vi "AO Post Step Type.vi"(8 "error in (no error)":errorcluster, 9 "AOWrite":T1, 10 "Socket No":u16=1, 11 "NI Analog Output in":refnum<class "NI Analog Output.lvclass">) -> (0 "error out":errorcluster, 2 "PhysicalChannel":string[](array[string]), 3 "NI Analog Output out":refnum<class "NI Analog Output.lvclass">)   [LabVIEW 2023, in "HardwareAbstractionLayer_LVOOP.lvlib" / "NI Analog Output.lvclass"]
uses:
  NI Analog Output.lvclass
  D:/eDCU LTT/VT LTT Project/Source Code/HardwareAbstractionLayer_LVOOP/Analog Output/AO/AO.lvclass
  NI Analog Output.lvclass/NI Analog Output.ctl
  Main/Class Options.ctl
  Main/Class Ref.ctl
  DMM/DMM.lvclass
  Function Generator/Function Generator.lvclass
  Oscilloscope/Oscilloscope.lvclass
  PowerSupply/PowerSupply.lvclass
  Teststand/Teststand.lvclass
  AO/AO.lvclass
  Analog Input/AI/AI.lvclass
  Database/Database.lvclass
  Digital Output/DO_class/DO.lvclass
  Digital Input/DI_class/DI.lvclass
  PWM Output/PWM Output_class/PWM Output.lvclass
  PWM Input/PWM Input_class/PWM Input.lvclass
  NI Switch/NISwitch_class/NISwitch.lvclass
  Modbus/Modbus_class/Modbus.lvclass
  CAN/CAN Lib/CAN_class/CAN.lvclass
  <resource>/objmgr/daqmx.rc
  Main/Main.lvclass
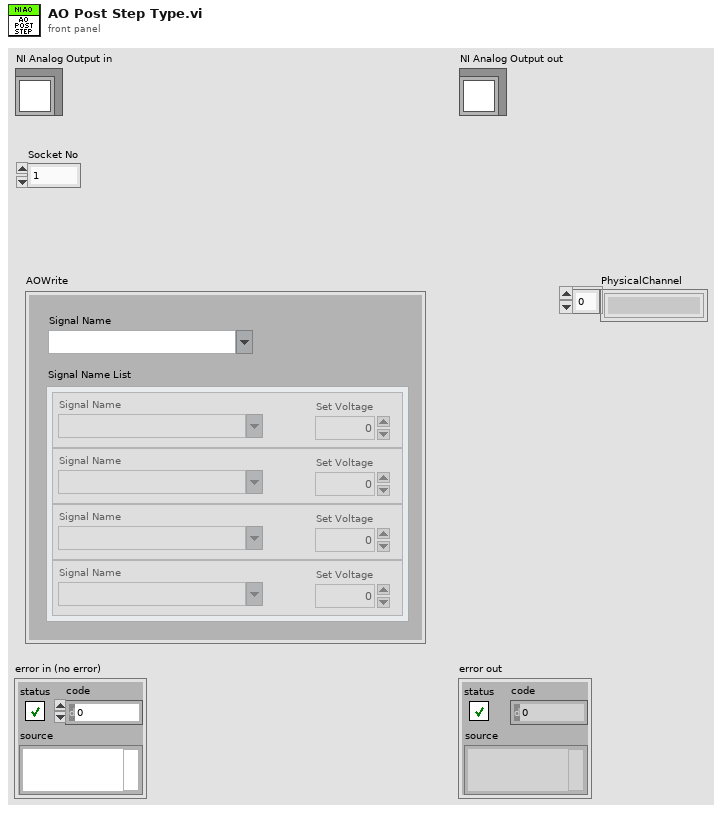
[diagram p1: front panel]
types:
  T1 = cluster{"Signal Name":string, "Signal Name List":cluster{"Signal Name":string, "Set Voltage":dbl}[]}
  T2 = typedef "HardwareAbstractionLayer_LVOOP.lvlib/Main.lvclass/Class Ref.ctl" = cluster{"DMM":refnum<class "DMM.lvclass">, "Function Generator":refnum<class "Function Generator.lvclass">, "Oscilloscope":refnum<class "Oscilloscope.lvclass">, "PowerSupply":refnum<class "PowerSupply.lvclass">, "Teststand":refnum<class "Teststand.lvclass">, "AO":refnum<class "AO.lvclass">, "AI":refnum<class "AI.lvclass">, "Database":refnum<class "Database.lvclass">, "AO Waveform Generation":refnum<class "AO.lvclass">, "DO":refnum<class "DO.lvclass">, "DI":refnum<class "DI.lvclass">, "PWM Output":refnum<class "PWM Output.lvclass">, "PWM Input":refnum<class "PWM Input.lvclass">, "RelayOutput":refnum<class "NISwitch.lvclass">, "Modbus":refnum<class "Modbus.lvclass">, "CAN":refnum<class "CAN.lvclass">}
  T3 = typedef "HardwareAbstractionLayer_LVOOP.lvlib/Main.lvclass/Class Options.ctl" = enum16{"Init All Class", "Read All Class", "Write AI Class", "Write AO Class", "Write AO Waveform Generation", "Write DI Class", "Write DO Class", "Write PWM Input Class", "Write PWM Output Class", "Exit"}
  T4 = cluster{"table":string, "condition":string, "columns":string[]}
  T5 = cluster{"Signal Name":string, "Set Voltage":dbl}[]
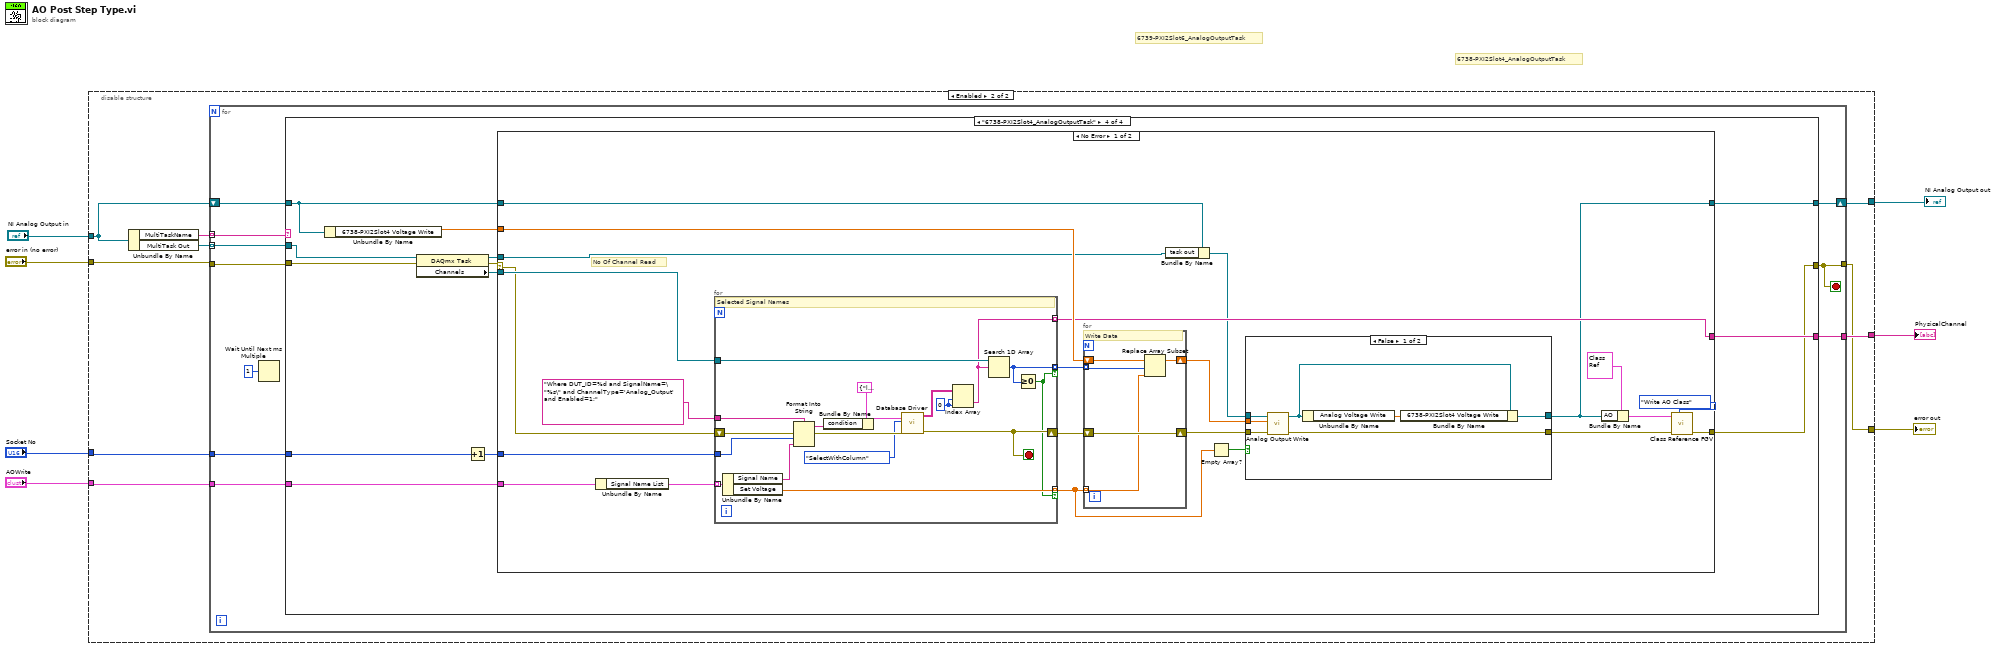
[diagram p0: block diagram]
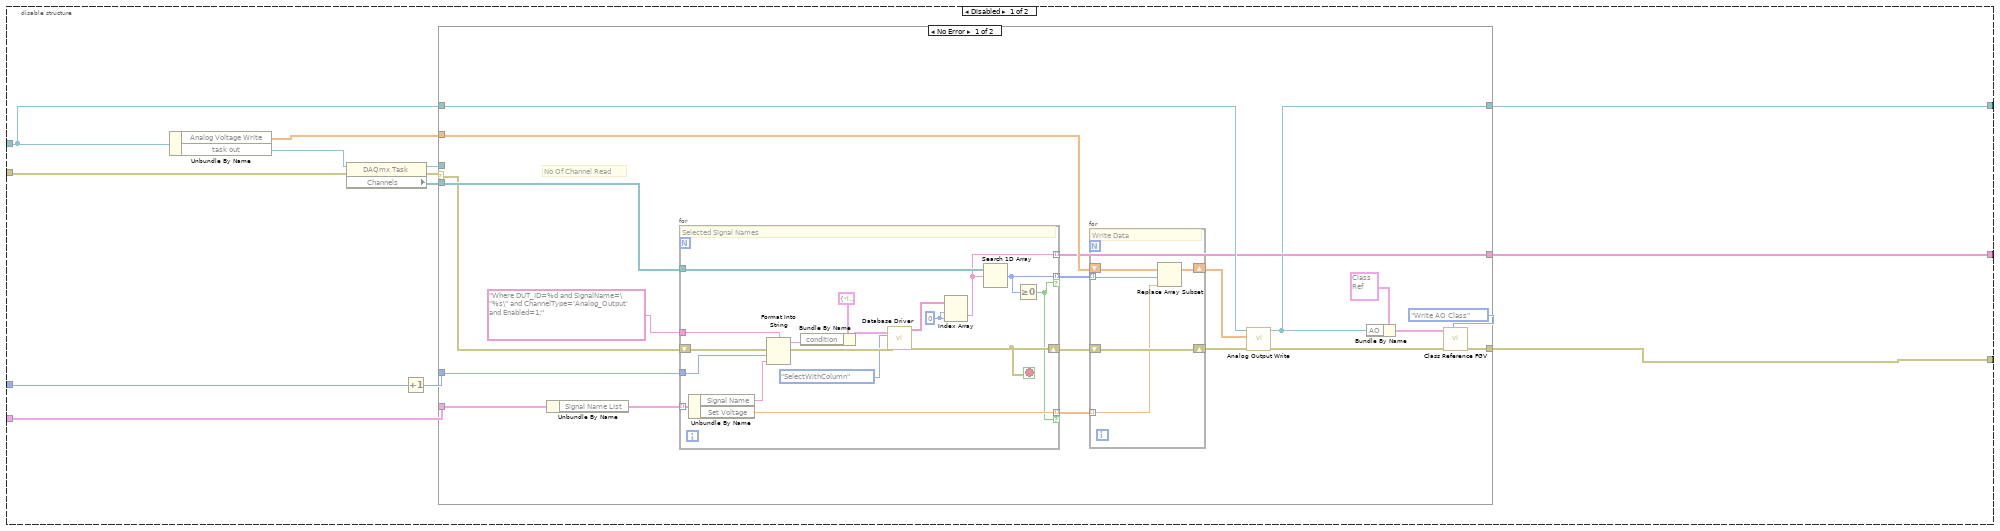
[diagram p2: hidden frame]
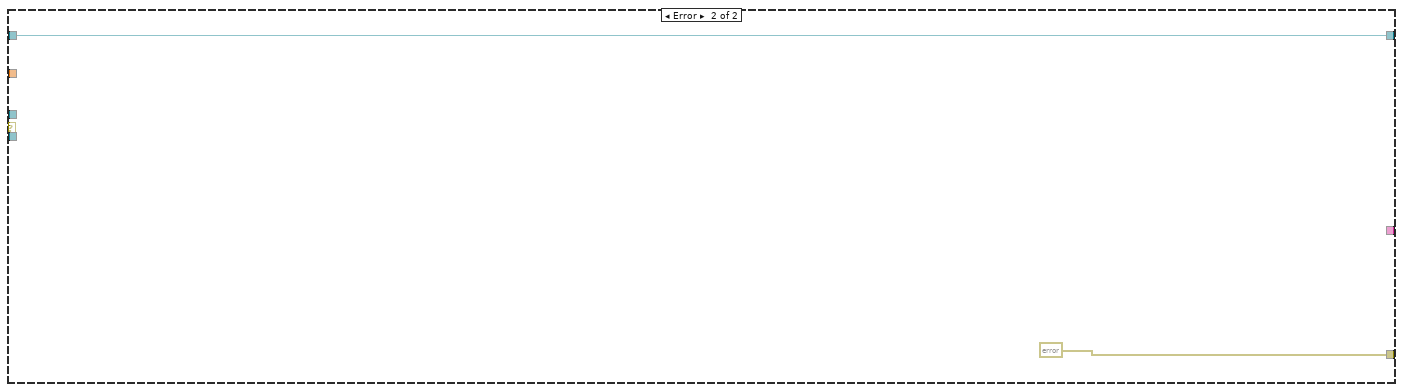
[diagram p3: hidden frame]
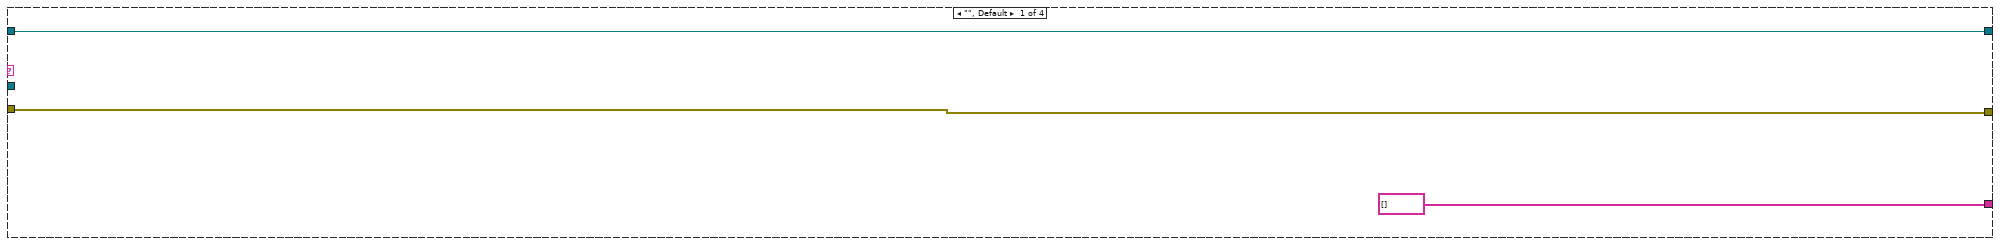
[diagram p4: hidden frame]
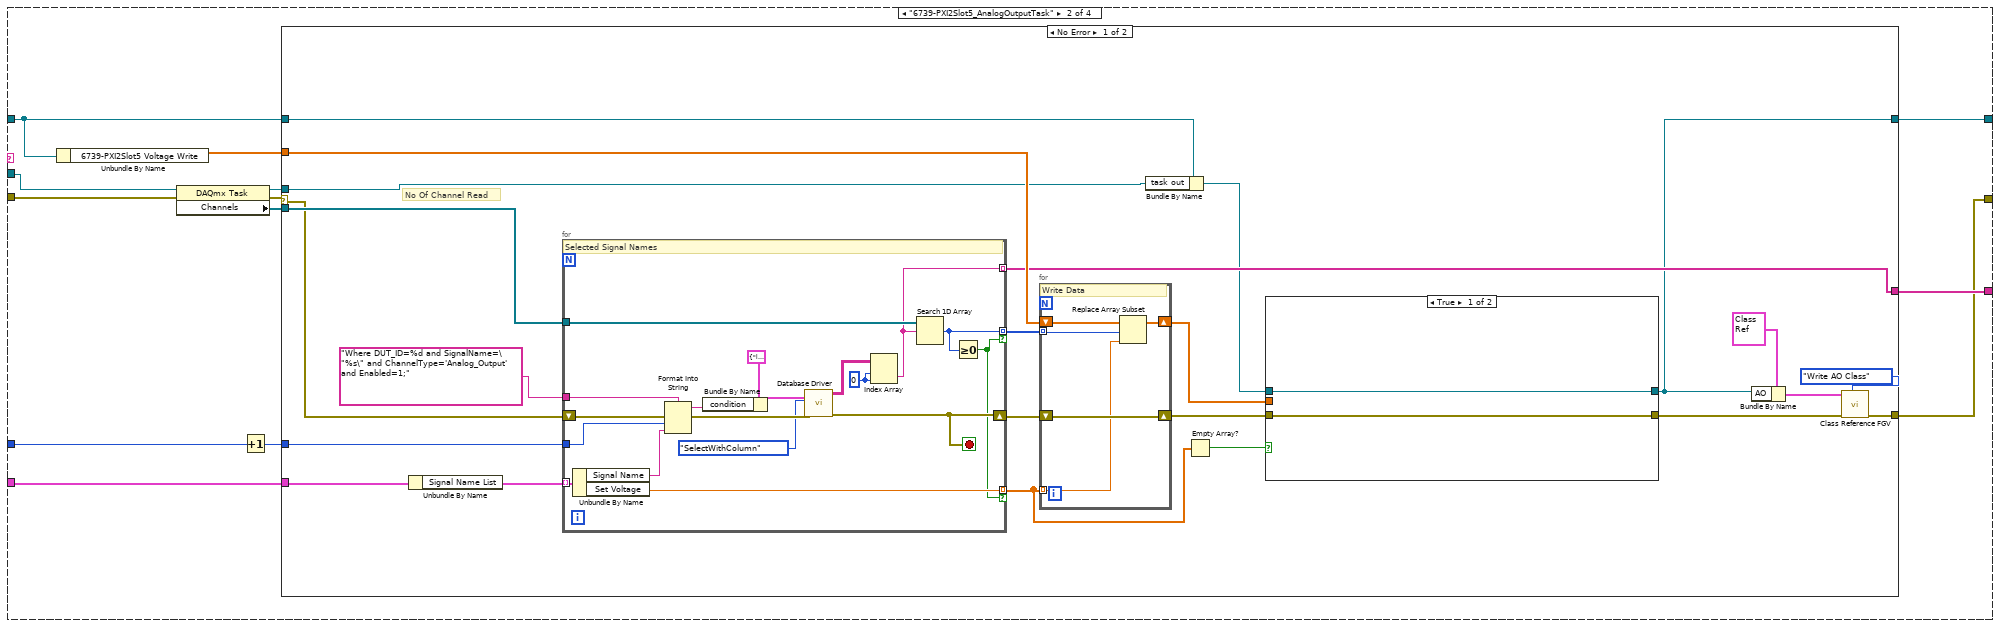
[diagram p5: hidden frame]
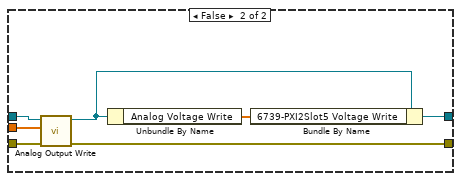
[diagram p6: hidden frame]
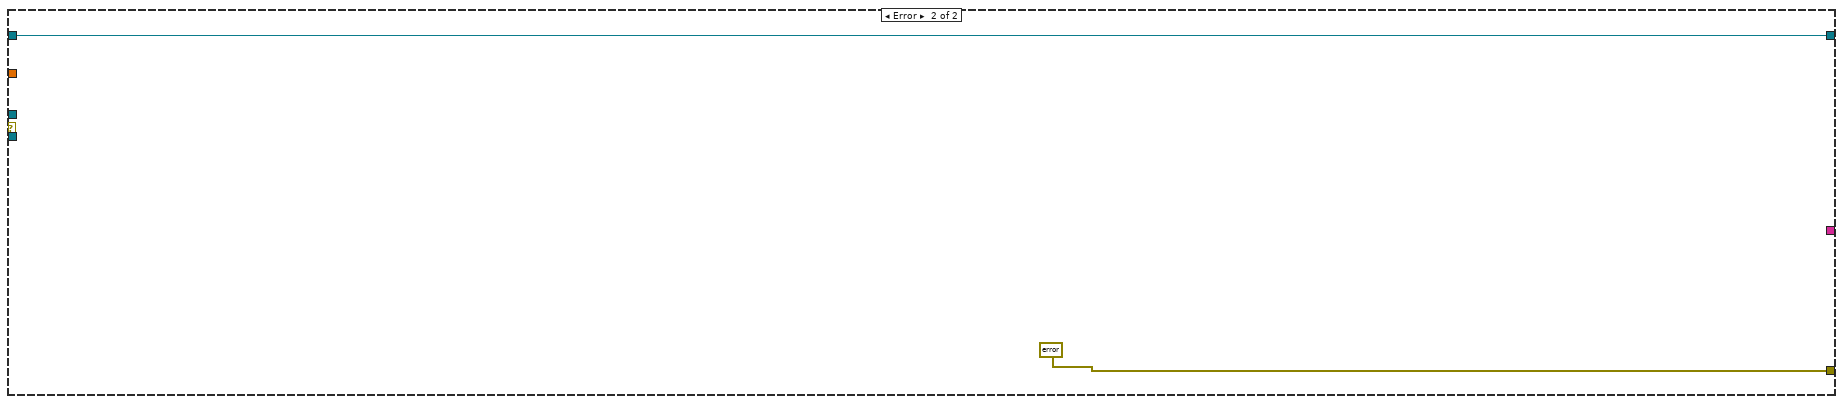
[diagram p7: hidden frame]
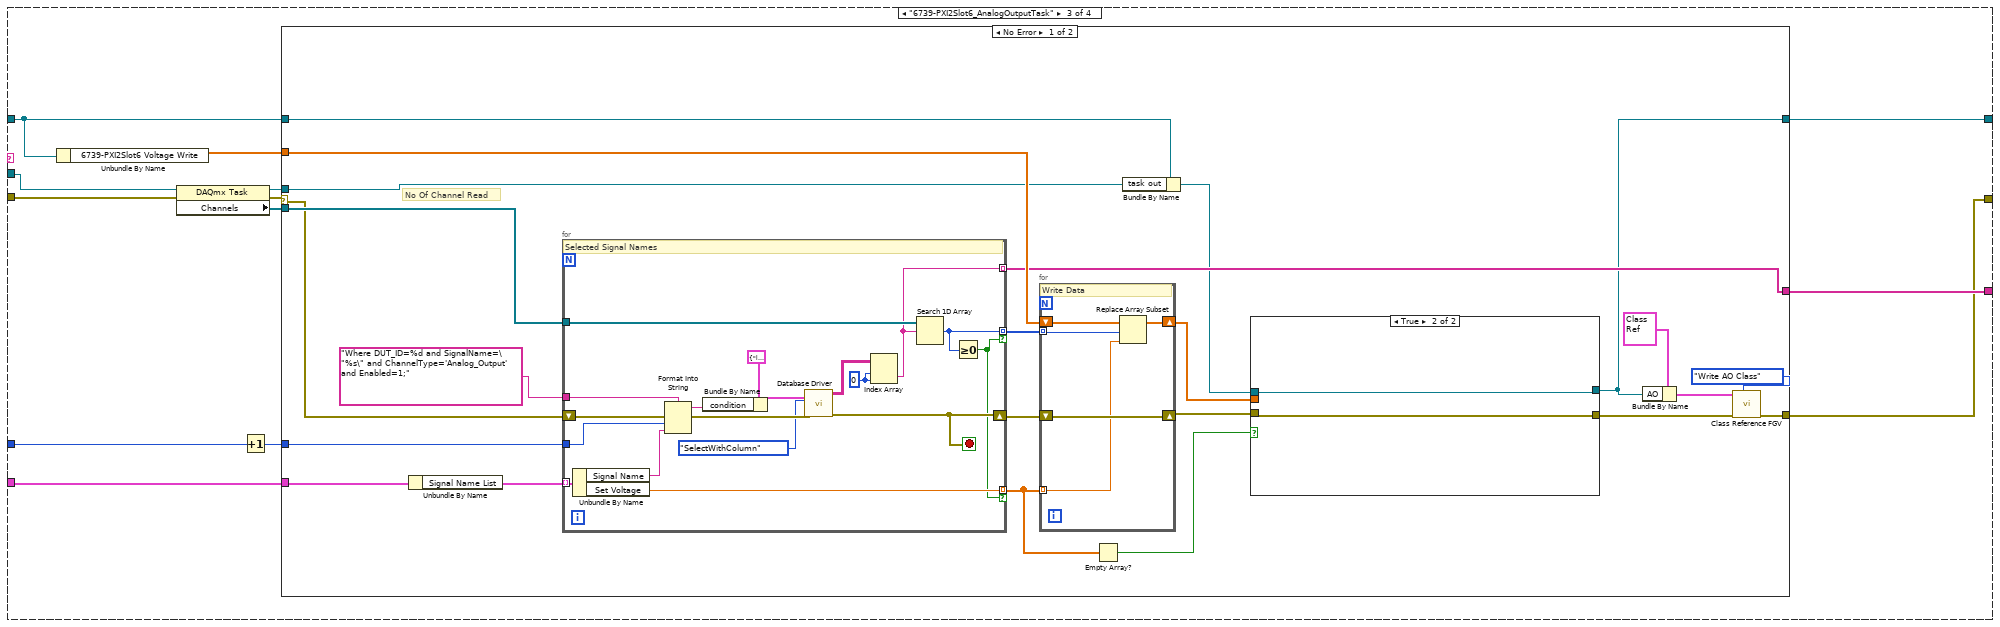
[diagram p8: hidden frame]
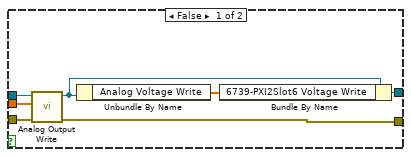
[diagram p9: hidden frame]
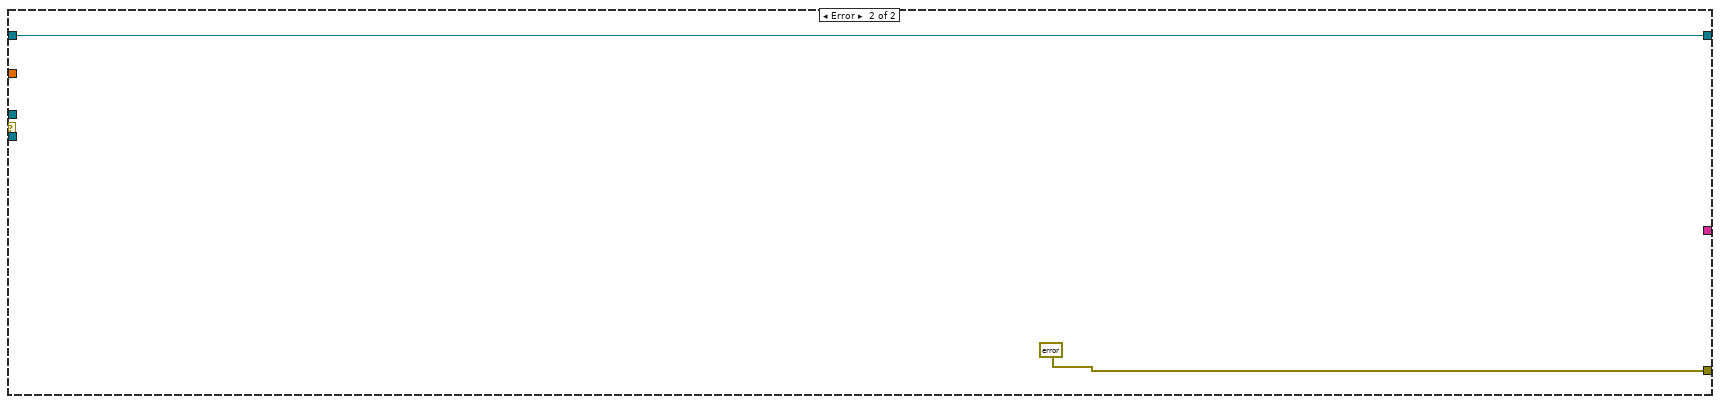
[diagram p10: hidden frame]
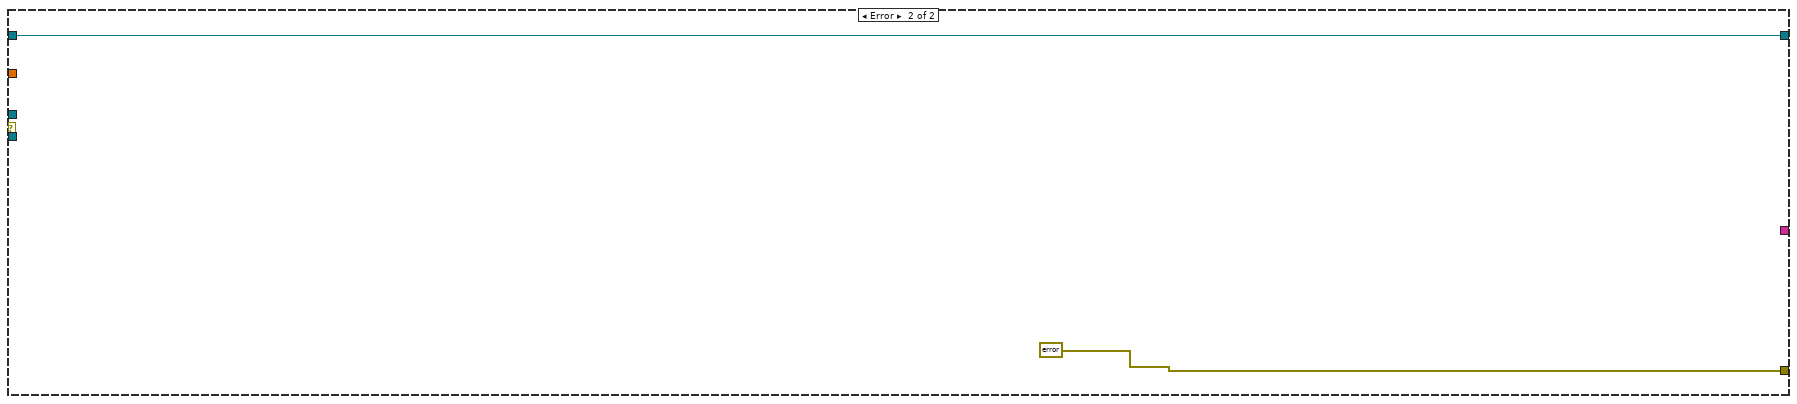
[diagram p12: hidden frame]
diagram:
  # "6738-PXI2Slot4_AnalogOutputTask"
  # "6739-PXI2Slot6_AnalogOutputTask"
  n1 = disable-structure shown="Enabled" {
    disable-tunnel: "AOWrite" -> [w19 w74]
    disable-tunnel: "Socket No" -> [w18 w73]
    disable-tunnel: "error in (no error)" -> [w14 w72]
    disable-tunnel: "NI Analog Output in" -> [w11 w68]
    disable-tunnel: [w10 w71] -> w3
    disable-tunnel: [w9 w70] -> w2
    disable-tunnel: [w8 w69] -> w1
    frame Disabled {
      n2 = Unbundle By Name(w11) -> ("Analog Voltage Write"=w12:dbl[], "task out"=w20:refnum<k21>)
      n3 = property class="DAQmx Task"(reference=w20, error in=w14) -> (reference out=w16:refnum<k21>, error out=w13:errorcluster, "Channels"=w15:refnum<k21>[])
      n4 = Increment(x=w18) -> (x+1=w17:u16)
      n5 = case shown="No Error" w13 {
        selector: w13 -> [w33 _]
        tunnel: [w24 errorcluster {"status"=TRUE, "code"=0, "source"="AO Task is not been created. please check in database."} ("error constant")] -> w8
        tunnel: w19 -> [w37 _]
        tunnel: w16 -> [_ _]
        tunnel: w15 -> [w35 _]
        tunnel: w17 -> [w34 _]
        tunnel: w12 -> [w31 _]
        tunnel: w11 -> [w30 w64]
        tunnel: [w21 w64] -> w10
        tunnel: [w27 _] -> w9
        frame No Error {
          # "No Of Channel Read"
          n6 = Unbundle By Name(w37) -> ("Signal Name List"=w40:T5)
          n7 = for {
            tunnel: w40 -> [w47] mode=indexing
            tunnel: "Where DUT_ID=%d and SignalName=\"%s\" and ChannelType='Analog_Output' and Enabled=1;" -> [w58]
            shift-right: [w49] -> w32
            shift-left: w33 -> [w54]
            tunnel: w35 -> [w43]
            tunnel: [w50] -> w38 mode=indexing if=w41
            tunnel: w34 -> [w48]
            tunnel: [w45] -> w36 mode=indexing if=w41
            tunnel: [w42] -> w27 mode=indexing
            stop <- w49 stop-if-true
            w51 = 0 ("disabled index (col)")
            # "Selected Signal Names"
            n8 = Unbundle By Name(w47) -> ("Signal Name"=w46:string, "Set Voltage"=w45:dbl)
            n9 = Format Into String(format string=w58, error in=w54, w48, w46) -> (resulting string=w56:string, error out=w53:errorcluster)  [unwired: 1 in]
            n10 = Bundle By Name(cluster=T4 {"table"="ltt.daq_configuration", "condition"="Where ChannelType='Analog_Input' and Enabled=1", "columns"=["PhysicalChannel"]} ("SQLTableData"), "condition"=w56) -> (w55:T4)
            n11 = call "Database Driver.vi"("SQLTableData"=w55, "error in"=w53, "Select"=enum16{"SelectWithQuery", "SelectWithColumn"}."SelectWithColumn") -> ("error out"=w49:errorcluster, "data"=w52:string[][])  [unwired: 5 in, 2 out]
            n12 = Index Array(array=w52, index (row)=w51, index (col)=w51) -> (element=w42:string)
            n13 = Search 1D Array(1D array=w43, element=w42) -> (index of element=w50:i32)  [unwired: 1 in]
            n14 = Greater Or Equal To 0?(x=w50) -> (x >= 0?=w41:bool)
          }
          n15 = for {
            shift-right: [w63] -> w29
            shift-left: w32 -> [w63]
            tunnel: w38 -> [w62] mode=indexing
            tunnel: w36 -> [w60] mode=indexing
            shift-right: [w59] -> w28
            shift-left: w31 -> [w61]
            # "Write Data"
            n16 = Replace Array Subset(array=w61, new element=w60, index=w62) -> (w59:dbl[])
          }
          n17 = call-dynamic "Analog Output Write.vi"("error in"=w29, "Analog Output Write"=w28, "NI Analog Output in"=w30) -> ("error out"=w25:errorcluster, "NI Analog Output out"=w21:refnum<class "NI Analog Output.lvclass">)  [unwired: 7 in]
          n18 = Bundle By Name(cluster=T2 {"DMM"=refnum, "Function Generator"=refnum, "Oscilloscope"=refnum, "PowerSupply"=refnum, "Teststand"=refnum, "AO"=refnum, "AI"=refnum, "Database"=refnum, "AO Waveform Generation"=refnum, "DO"=refnum, "DI"=refnum, "PWM Output"=refnum, "PWM Input"=refnum, "RelayOutput"=refnum, "Modbus"=refnum, "CAN"=refnum} ("Class Cluster In"), "AO"=w21) -> (w22:T2)
          n19 = call "Class Reference FGV.vi"("Options"=Class_Options."Write AO Class", "error in"=w25, "Class Cluster In"=w22) -> ("error out"=w24:errorcluster)  [unwired: 7 in, 1 out]
        }
        frame Error {
        }
      }
    }
    frame Enabled {
      n20 = Unbundle By Name(w68) -> ("MultiTaskName"=w67:string[], "MultiTask Out"=w66:refnum<k21>[])
      n21 = for {
        tunnel: w74 -> [w84]
        tunnel: w73 -> [w83]
        tunnel: [w80] -> w70
        shift-right: [w81] -> w71
        shift-left: w68 -> [w79]
        tunnel: w67 -> [w77] mode=indexing
        tunnel: w66 -> [w76] mode=indexing
        tunnel: w72 -> [w82]
        tunnel: [w78] -> w69
        stop <- w78 stop-if-true
        n22 = Wait Until Next ms Multiple(millisecond multiple=u32 1) -> ()  [unwired: 1 out]
        n23 = case shown="\"6738-PXI2Slot4_AnalogOutputTask\"" w77 {
          tunnel: w84 -> [_ w95 w165 w235]
          tunnel: w83 -> [_ w94 w164 w234]
          tunnel: w82 -> [w86 w93 w163 w233]
          tunnel: [w87 w92 w162 w232] -> w81
          tunnel: [string[] [] w91 w161 w231] -> w80
          tunnel: w79 -> [w87 w89 w159 w229]
          tunnel: [w86 w90 w160 w230] -> w78
          tunnel: w76 -> [_ w88 w158 w228]
          frame "", Default {
          }
          frame "6739-PXI2Slot5_AnalogOutputTask" {
            n24 = Unbundle By Name(w89) -> ("6739-PXI2Slot5 Voltage Write"=w96:dbl[])
            n25 = property class="DAQmx Task"(reference=w88, error in=w93) -> (reference out=w99:refnum<k21>, error out=w97:errorcluster, "Channels"=w98:refnum<k21>[])
            n26 = Increment(x=w94) -> (x+1=w100:u16)
            n27 = case shown="No Error" w97 {
              selector: w97 -> [w117 _]
              tunnel: [w110 errorcluster {"status"=TRUE, "code"=0, "source"="AO Task is not been created. please check in database."} ("error constant")] -> w90
              tunnel: w95 -> [w120 _]
              tunnel: w99 -> [w106 _]
              tunnel: w98 -> [w119 _]
              tunnel: w100 -> [w118 _]
              tunnel: w96 -> [w115 _]
              tunnel: w89 -> [w104 w156]
              tunnel: [w103 w156] -> w92
              tunnel: [w113 _] -> w91
              frame No Error {
                # "No Of Channel Read"
                n28 = Unbundle By Name(w120) -> ("Signal Name List"=w123:T5)
                n29 = for {
                  tunnel: w123 -> [w139] mode=indexing
                  tunnel: "Where DUT_ID=%d and SignalName=\"%s\" and ChannelType='Analog_Output' and Enabled=1;" -> [w150]
                  shift-right: [w141] -> w116
                  shift-left: w117 -> [w146]
                  tunnel: w119 -> [w135]
                  tunnel: [w142] -> w121 mode=indexing if=w133
                  tunnel: w118 -> [w140]
                  tunnel: [w137] -> w102 mode=indexing if=w133
                  tunnel: [w134] -> w113 mode=indexing
                  stop <- w141 stop-if-true
                  w143 = 0 ("disabled index (col)")
                  # "Selected Signal Names"
                  n30 = Unbundle By Name(w139) -> ("Signal Name"=w138:string, "Set Voltage"=w137:dbl)
                  n31 = Format Into String(format string=w150, error in=w146, w140, w138) -> (resulting string=w148:string, error out=w145:errorcluster)  [unwired: 1 in]
                  n32 = Bundle By Name(cluster=T4 {"table"="ltt.daq_configuration", "condition"="Where ChannelType='Analog_Input' and Enabled=1", "columns"=["PhysicalChannel"]} ("SQLTableData"), "condition"=w148) -> (w147:T4)
                  n33 = call "Database Driver.vi"("SQLTableData"=w147, "error in"=w145, "Select"=enum16{"SelectWithQuery", "SelectWithColumn"}."SelectWithColumn") -> ("error out"=w141:errorcluster, "data"=w144:string[][])  [unwired: 5 in, 2 out]
                  n34 = Index Array(array=w144, index (row)=w143, index (col)=w143) -> (element=w134:string)
                  n35 = Search 1D Array(1D array=w135, element=w134) -> (index of element=w142:i32)  [unwired: 1 in]
                  n36 = Greater Or Equal To 0?(x=w142) -> (x >= 0?=w133:bool)
                }
                n37 = for {
                  shift-right: [w155] -> w114
                  shift-left: w116 -> [w155]
                  tunnel: w121 -> [w154] mode=indexing
                  tunnel: w102 -> [w151] mode=indexing
                  shift-right: [w152] -> w107
                  shift-left: w115 -> [w153]
                  # "Write Data"
                  n38 = Replace Array Subset(array=w153, new element=w151, index=w154) -> (w152:dbl[])
                }
                n39 = Bundle By Name(cluster=w104, "task out"=w106) -> (w105:refnum<class "NI Analog Output.lvclass">)
                n40 = Empty Array?(array=w102) -> (empty?=w101:bool)
                n41 = case shown="True" w101 {
                  tunnel: w114 -> [w125 w132]
                  tunnel: [w125 w131] -> w111
                  tunnel: w107 -> [_ w130]
                  tunnel: w105 -> [w124 w129]
                  tunnel: [w124 w126] -> w103
                  frame True {
                  }
                  frame False {
                    n42 = call-dynamic "Analog Output Write.vi"("error in"=w132, "Analog Output Write"=w130, "NI Analog Output in"=w129) -> ("error out"=w131:errorcluster, "NI Analog Output out"=w128:refnum<class "NI Analog Output.lvclass">)  [unwired: 7 in]
                    n43 = Unbundle By Name(w128) -> ("Analog Voltage Write"=w127:dbl[])
                    n44 = Bundle By Name(cluster=w128, "6739-PXI2Slot5 Voltage Write"=w127) -> (w126:refnum<class "NI Analog Output.lvclass">)
                  }
                }
                n45 = Bundle By Name(cluster=T2 {"DMM"=refnum, "Function Generator"=refnum, "Oscilloscope"=refnum, "PowerSupply"=refnum, "Teststand"=refnum, "AO"=refnum, "AI"=refnum, "Database"=refnum, "AO Waveform Generation"=refnum, "DO"=refnum, "DI"=refnum, "PWM Output"=refnum, "PWM Input"=refnum, "RelayOutput"=refnum, "Modbus"=refnum, "CAN"=refnum} ("Class Cluster In"), "AO"=w103) -> (w108:T2)
                n46 = call "Class Reference FGV.vi"("Options"=Class_Options."Write AO Class", "error in"=w111, "Class Cluster In"=w108) -> ("error out"=w110:errorcluster)  [unwired: 7 in, 1 out]
              }
              frame Error {
              }
            }
          }
          frame "6739-PXI2Slot6_AnalogOutputTask" {
            n47 = Unbundle By Name(w159) -> ("6739-PXI2Slot6 Voltage Write"=w166:dbl[])
            n48 = property class="DAQmx Task"(reference=w158, error in=w163) -> (reference out=w169:refnum<k21>, error out=w167:errorcluster, "Channels"=w168:refnum<k21>[])
            n49 = Increment(x=w164) -> (x+1=w170:u16)
            n50 = case shown="No Error" w167 {
              selector: w167 -> [w187 _]
              tunnel: [w180 errorcluster {"status"=TRUE, "code"=0, "source"="AO Task is not been created. please check in database."} ("error constant")] -> w160
              tunnel: w165 -> [w190 _]
              tunnel: w169 -> [w176 _]
              tunnel: w168 -> [w189 _]
              tunnel: w170 -> [w188 _]
              tunnel: w166 -> [w185 _]
              tunnel: w159 -> [w174 w226]
              tunnel: [w173 w226] -> w162
              tunnel: [w183 _] -> w161
              frame No Error {
                # "No Of Channel Read"
                n51 = Unbundle By Name(w190) -> ("Signal Name List"=w193:T5)
                n52 = for {
                  tunnel: w193 -> [w209] mode=indexing
                  tunnel: "Where DUT_ID=%d and SignalName=\"%s\" and ChannelType='Analog_Output' and Enabled=1;" -> [w220]
                  shift-right: [w211] -> w186
                  shift-left: w187 -> [w216]
                  tunnel: w189 -> [w205]
                  tunnel: [w212] -> w191 mode=indexing if=w203
                  tunnel: w188 -> [w210]
                  tunnel: [w207] -> w172 mode=indexing if=w203
                  tunnel: [w204] -> w183 mode=indexing
                  stop <- w211 stop-if-true
                  w213 = 0 ("disabled index (col)")
                  # "Selected Signal Names"
                  n53 = Unbundle By Name(w209) -> ("Signal Name"=w208:string, "Set Voltage"=w207:dbl)
                  n54 = Format Into String(format string=w220, error in=w216, w210, w208) -> (resulting string=w218:string, error out=w215:errorcluster)  [unwired: 1 in]
                  n55 = Bundle By Name(cluster=T4 {"table"="ltt.daq_configuration", "condition"="Where ChannelType='Analog_Input' and Enabled=1", "columns"=["PhysicalChannel"]} ("SQLTableData"), "condition"=w218) -> (w217:T4)
                  n56 = call "Database Driver.vi"("SQLTableData"=w217, "error in"=w215, "Select"=enum16{"SelectWithQuery", "SelectWithColumn"}."SelectWithColumn") -> ("error out"=w211:errorcluster, "data"=w214:string[][])  [unwired: 5 in, 2 out]
                  n57 = Index Array(array=w214, index (row)=w213, index (col)=w213) -> (element=w204:string)
                  n58 = Search 1D Array(1D array=w205, element=w204) -> (index of element=w212:i32)  [unwired: 1 in]
                  n59 = Greater Or Equal To 0?(x=w212) -> (x >= 0?=w203:bool)
                }
                n60 = for {
                  shift-right: [w225] -> w184
                  shift-left: w186 -> [w225]
                  tunnel: w191 -> [w224] mode=indexing
                  tunnel: w172 -> [w221] mode=indexing
                  shift-right: [w222] -> w177
                  shift-left: w185 -> [w223]
                  # "Write Data"
                  n61 = Replace Array Subset(array=w223, new element=w221, index=w224) -> (w222:dbl[])
                }
                n62 = Empty Array?(array=w172) -> (empty?=w171:bool)
                n63 = Bundle By Name(cluster=w174, "task out"=w176) -> (w175:refnum<class "NI Analog Output.lvclass">)
                n64 = case shown="True" w171 {
                  tunnel: w184 -> [w200 w201]
                  tunnel: [w199 w201] -> w181
                  tunnel: w177 -> [w198 _]
                  tunnel: w175 -> [w197 w202]
                  tunnel: [w194 w202] -> w173
                  frame False {
                    n65 = call-dynamic "Analog Output Write.vi"("error in"=w200, "Analog Output Write"=w198, "NI Analog Output in"=w197) -> ("error out"=w199:errorcluster, "NI Analog Output out"=w196:refnum<class "NI Analog Output.lvclass">)  [unwired: 7 in]
                    n66 = Unbundle By Name(w196) -> ("Analog Voltage Write"=w195:dbl[])
                    n67 = Bundle By Name(cluster=w196, "6739-PXI2Slot6 Voltage Write"=w195) -> (w194:refnum<class "NI Analog Output.lvclass">)
                  }
                  frame True {
                  }
                }
                n68 = Bundle By Name(cluster=T2 {"DMM"=refnum, "Function Generator"=refnum, "Oscilloscope"=refnum, "PowerSupply"=refnum, "Teststand"=refnum, "AO"=refnum, "AI"=refnum, "Database"=refnum, "AO Waveform Generation"=refnum, "DO"=refnum, "DI"=refnum, "PWM Output"=refnum, "PWM Input"=refnum, "RelayOutput"=refnum, "Modbus"=refnum, "CAN"=refnum} ("Class Cluster In"), "AO"=w173) -> (w178:T2)
                n69 = call "Class Reference FGV.vi"("Options"=Class_Options."Write AO Class", "error in"=w181, "Class Cluster In"=w178) -> ("error out"=w180:errorcluster)  [unwired: 7 in, 1 out]
              }
              frame Error {
              }
            }
          }
          frame "6738-PXI2Slot4_AnalogOutputTask" {
            n70 = Unbundle By Name(w229) -> ("6738-PXI2Slot4 Voltage Write"=w236:dbl[])
            n71 = property class="DAQmx Task"(reference=w228, error in=w233) -> (reference out=w239:refnum<k21>, error out=w237:errorcluster, "Channels"=w238:refnum<k21>[])
            n72 = Increment(x=w234) -> (x+1=w240:u16)
            n73 = case shown="No Error" w237 {
              selector: w237 -> [w257 _]
              tunnel: [w250 errorcluster {"status"=TRUE, "code"=0, "source"="AO Task is not been created. please check in database."} ("error constant")] -> w230
              tunnel: w235 -> [w260 _]
              tunnel: w239 -> [w246 _]
              tunnel: w238 -> [w259 _]
              tunnel: w240 -> [w258 _]
              tunnel: w236 -> [w255 _]
              tunnel: w229 -> [w244 w296]
              tunnel: [w243 w296] -> w232
              tunnel: [w253 _] -> w231
              frame No Error {
                # "No Of Channel Read"
                n74 = Unbundle By Name(w260) -> ("Signal Name List"=w263:T5)
                n75 = for {
                  tunnel: w263 -> [w279] mode=indexing
                  tunnel: "Where DUT_ID=%d and SignalName=\"%s\" and ChannelType='Analog_Output' and Enabled=1;" -> [w290]
                  shift-right: [w281] -> w256
                  shift-left: w257 -> [w286]
                  tunnel: w259 -> [w275]
                  tunnel: [w282] -> w261 mode=indexing if=w273
                  tunnel: w258 -> [w280]
                  tunnel: [w277] -> w242 mode=indexing if=w273
                  tunnel: [w274] -> w253 mode=indexing
                  stop <- w281 stop-if-true
                  w283 = 0 ("disabled index (col)")
                  # "Selected Signal Names"
                  n76 = Unbundle By Name(w279) -> ("Signal Name"=w278:string, "Set Voltage"=w277:dbl)
                  n77 = Format Into String(format string=w290, error in=w286, w280, w278) -> (resulting string=w288:string, error out=w285:errorcluster)  [unwired: 1 in]
                  n78 = Bundle By Name(cluster=T4 {"table"="ltt.daq_configuration", "condition"="Where ChannelType='Analog_Input' and Enabled=1", "columns"=["PhysicalChannel"]} ("SQLTableData"), "condition"=w288) -> (w287:T4)
                  n79 = call "Database Driver.vi"("SQLTableData"=w287, "error in"=w285, "Select"=enum16{"SelectWithQuery", "SelectWithColumn"}."SelectWithColumn") -> ("error out"=w281:errorcluster, "data"=w284:string[][])  [unwired: 5 in, 2 out]
                  n80 = Index Array(array=w284, index (row)=w283, index (col)=w283) -> (element=w274:string)
                  n81 = Search 1D Array(1D array=w275, element=w274) -> (index of element=w282:i32)  [unwired: 1 in]
                  n82 = Greater Or Equal To 0?(x=w282) -> (x >= 0?=w273:bool)
                }
                n83 = for {
                  shift-right: [w295] -> w254
                  shift-left: w256 -> [w295]
                  tunnel: w261 -> [w294] mode=indexing
                  tunnel: w242 -> [w291] mode=indexing
                  shift-right: [w292] -> w247
                  shift-left: w255 -> [w293]
                  # "Write Data"
                  n84 = Replace Array Subset(array=w293, new element=w291, index=w294) -> (w292:dbl[])
                }
                n85 = Bundle By Name(cluster=w244, "task out"=w246) -> (w245:refnum<class "NI Analog Output.lvclass">)
                n86 = Empty Array?(array=w242) -> (empty?=w241:bool)
                n87 = case shown="False" w241 {
                  tunnel: w254 -> [w270 w271]
                  tunnel: [w269 w271] -> w251
                  tunnel: w247 -> [w268 _]
                  tunnel: w245 -> [w267 w272]
                  tunnel: [w264 w272] -> w243
                  frame False {
                    n88 = call-dynamic "Analog Output Write.vi"("error in"=w270, "Analog Output Write"=w268, "NI Analog Output in"=w267) -> ("error out"=w269:errorcluster, "NI Analog Output out"=w266:refnum<class "NI Analog Output.lvclass">)  [unwired: 7 in]
                    n89 = Unbundle By Name(w266) -> ("Analog Voltage Write"=w265:dbl[])
                    n90 = Bundle By Name(cluster=w266, "6738-PXI2Slot4 Voltage Write"=w265) -> (w264:refnum<class "NI Analog Output.lvclass">)
                  }
                  frame True {
                  }
                }
                n91 = Bundle By Name(cluster=T2 {"DMM"=refnum, "Function Generator"=refnum, "Oscilloscope"=refnum, "PowerSupply"=refnum, "Teststand"=refnum, "AO"=refnum, "AI"=refnum, "Database"=refnum, "AO Waveform Generation"=refnum, "DO"=refnum, "DI"=refnum, "PWM Output"=refnum, "PWM Input"=refnum, "RelayOutput"=refnum, "Modbus"=refnum, "CAN"=refnum} ("Class Cluster In"), "AO"=w243) -> (w248:T2)
                n92 = call "Class Reference FGV.vi"("Options"=Class_Options."Write AO Class", "error in"=w251, "Class Cluster In"=w248) -> ("error out"=w250:errorcluster)  [unwired: 7 in, 1 out]
              }
              frame Error {
              }
            }
          }
        }
      }
    }
  }
  "error out" <- w1
  "NI Analog Output out" <- w3
  "PhysicalChannel" <- w2
